vi "Arrow.vi"() -> ()   [LabVIEW 2018]
panel:
  out "칸수":dbl
  in  "층":dbl
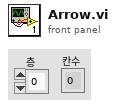
[diagram p1: front panel]
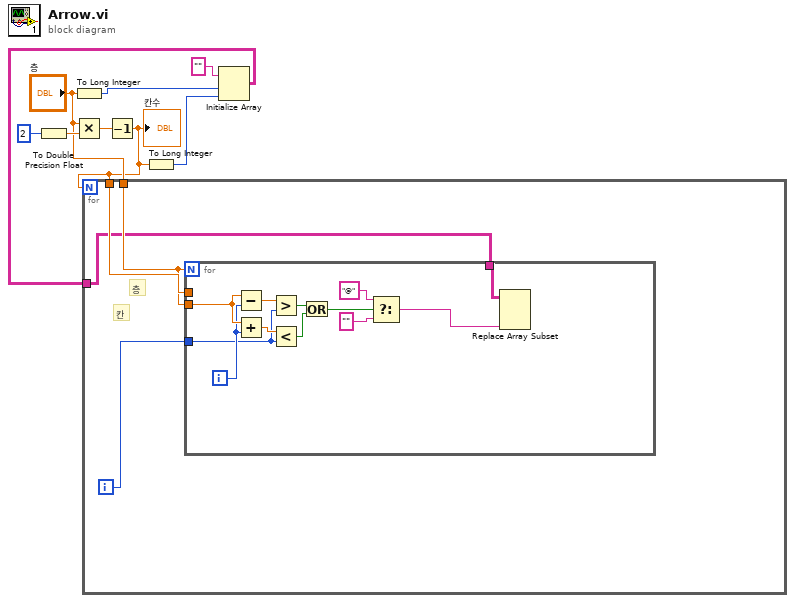
[diagram p0: block diagram]
diagram:
  n1 = To Double Precision Float(number=2) -> (double precision float=w7:dbl)
  n2 = To Long Integer(number="층") -> (32bit integer=w3:i32)
  n3 = Multiply(x="층", y=w7) -> (x*y=w8:dbl)
  n4 = Decrement(x=w8) -> (x-1=w1:dbl)
  "칸수" <- w1
  n5 = To Long Integer(number=w1) -> (32bit integer=w4:i32)
  n6 = Initialize Array("", w3, w4) -> (w6:string[][])
  n7 = for {
    N: w1 -> [_]
    tunnel: w6 -> [w10]
    tunnel: "층" -> [w12]
    tunnel: w1 -> [w13]
    i -> [w11]
    # "층"
    # "칸"
    n8 = for {
      N: w12 -> [_]
      tunnel: w13 -> [_]
      tunnel: w12 -> [w23]
      tunnel: w11 -> [w15]
      tunnel: w10 -> [w16]
      i -> [w22]
      n9 = Subtract(x=w23, y=w22) -> (x-y=w21:dbl)
      n10 = Add(x=w23, y=w22) -> (x+y=w20:dbl)
      n11 = Greater?(x=w21, y=w15) -> (0:w25:bool)
      n12 = Less?(x=w20, y=w15) -> (x < y?=w24:bool)
      n13 = Or(x=w25, y=w24) -> (x .or. y?=w19:bool)
      n14 = Select(t="@", s=w19, f="") -> (s? t:f=w14:string)
      n15 = Replace Array Subset(array=w16, new element=w14) -> ()  [unwired: 2 in, 1 out]
    }
  }
